vi "Up Vector Check.vi"(8 "Column":i32, 9 "Row":i32, 10 "Opponent's Tiles":bool[][](array[boolean]), 11 "Current Player's Tiles":bool[][](array[boolean])) -> (2 "Possible Flips":T1[](array[typedef]), 3 "Possible Location":bool)   [LabVIEW 2020, in "Reversi.lvlib" / "Reversi.lvclass"]
uses:
  Reversi.lvclass
  Space Coordinates.ctl
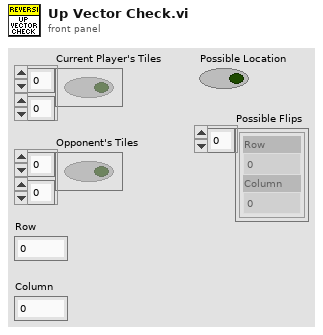
[diagram p1: front panel]
types:
  T1 = typedef "Reversi.lvlib/Reversi.lvclass/Space Coordinates.ctl" = cluster{"Row":i32, "Column":i32}
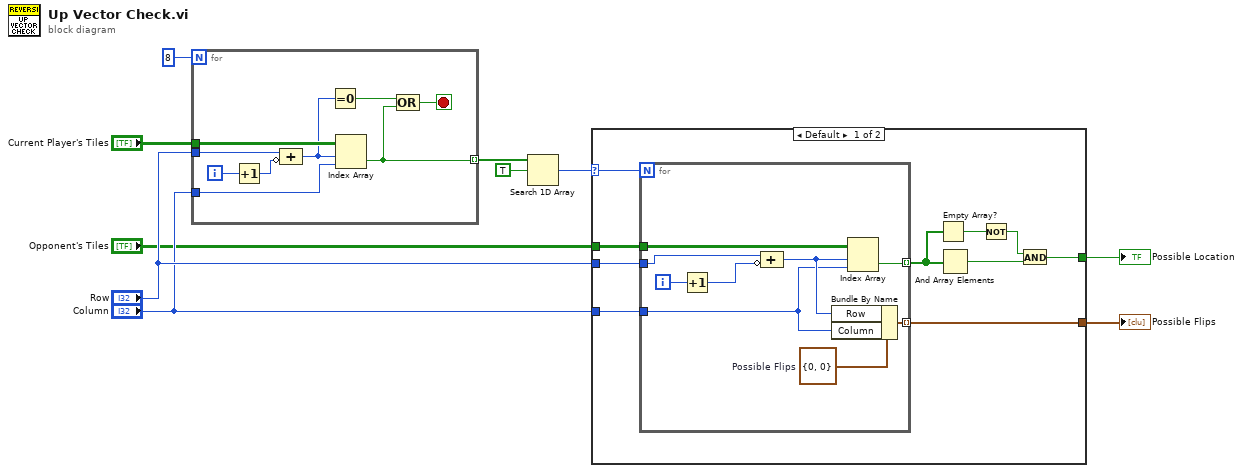
[diagram p0: block diagram]
diagram:
  n1 = for {
    N: 8 -> [_]
    tunnel: [w13] -> w9 mode=indexing
    tunnel: "Current Player's Tiles" -> [w19]
    tunnel: "Column" -> [w11]
    tunnel: "Row" -> [w17]
    i -> [w18]
    stop <- w12 stop-if-true
    n2 = Increment(x=w18) -> (x+1=w16:i32)
    n3 = Compound Arithmetic op=ADD(w17, invert w16) -> (w15:i32)
    n4 = Equal To 0?(x=w15) -> (x = 0?=w14:bool)
    n5 = Index Array(array=w19, index (row)=w15, index (col)=w11) -> (element=w13:bool)
    n6 = Compound Arithmetic op=OR(w14, w13) -> (w12:bool)
  }
  n7 = Search 1D Array(1D array=w9, element=TRUE) -> (index of element=w2:i32)  [unwired: 1 in]
  n8 = case shown="Default" w2 {
    selector: w2 -> [w20 _]
    tunnel: "Opponent's Tiles" -> [w25 _]
    tunnel: "Column" -> [w23 _]
    tunnel: [w26 _] -> w6
    tunnel: "Row" -> [w24 _]
    tunnel: [w21 _] -> w10
    frame Default {
      n9 = for {
        N: w20 -> [_]
        tunnel: [w36] -> w22 mode=indexing
        tunnel: w25 -> [w38]
        tunnel: w24 -> [w34]
        tunnel: w23 -> [w31]
        tunnel: [w33] -> w21 mode=indexing
        i -> [w37]
        w30 = T1 {"Row"=0, "Column"=0}  # Possible Flips
        n10 = Increment(x=w37) -> (x+1=w35:i32)
        n11 = Compound Arithmetic op=ADD(w34, invert w35) -> (w32:i32)
        n12 = Bundle By Name(cluster=w30, "Row"=w32, "Column"=w31) -> (w33:T1)
        n13 = Index Array(array=w38, index (row)=w32, index (col)=w31) -> (element=w36:bool)
      }
      n14 = Empty Array?(array=w22) -> (empty?=w29:bool)
      n15 = And Array Elements(Boolean array=w22) -> (logical AND=w27:bool)
      n16 = Not(x=w29) -> (.not. x?=w28:bool)
      n17 = And(x=w28, y=w27) -> (x .and. y?=w26:bool)
    }
    frame -1 {
    }
  }
  "Possible Flips" <- w10
  "Possible Location" <- w6
